vi "Cuadricula.vi"(0 "Image In":T3, 1 "ROI Descriptor (Pattern Matching 1)":T2={"Global Rectangle"=[20, 20, 1260, 700], "Contours"=[{"ID"=enum."External", "Type"=3, "Coordinates"=[20, 20, 1260, 700]}]} {"Contours"."Type" items=["No Selection", "Point", "Line", "Rectangle", "Oval", "Polygon", "Freehand Region", "Annulus", "Unused2", "Unused3", "Broken Line", "Freehand Line", "Rotated Rectangle"]}, 2 "Advanced Options (Pattern Matching 1)":cluster{"Item":T1, "Value":dbl}[](array[cluster]) {"Item" items=["LD Sampling - Minimum Constrast"=0, "LD Sampling - Enable Subpixel Accuracy"=1, "LD Sampling - Search Strategy"=2, "LD Sampling - Subpixel Iterations"=3, "LD Sampling - Subpixel Tolerance"=4, "LD Sampling - Initial Match List Length"=5, "LD Sampling - Match List Reduction Factor"=6, "LD Sampling - Initial Step Size"=7, "LD Sampling - Intermediate Angular Accuracy"=8, "-"=9, "Pyramid - Max Pyramid Level"=100, "Pyramid - Minimum Contrast"=102, "Pyramid - Enable Subpixel Accuracy"=103, "Pyramid - Subpixel Iterations"=104, "Pyramid - Subpixel Tolerance"=105, "Pyramid - Initial Match List Length"=106, "Pyramid - Match List Reduction Factor"=107, "Pyramid - Intermediate Angular Accuracy"=108, "Pyramid - Process Border Matches"=109, "Pyramid - Min Match Separation Distance"=111, "Pyramid - Min Match Separation Angle"=112, "Pyramid - Max Match Overlap"=113, "Pyramid - Max Cache in MB"=114, "Pyramid - Clear Cache"=115, "Pyramid - Enable Accurate Score Computation"=116, "Pyramid - Interpolation Method For Score Computation"=117, "Pyramid - Enable Target To Template Score"=118, "-"=119, "Enable Defect Map"=200]}, 3 "Template File Path (Pattern Matching 1)":path=path "C:/Users/cseba/OneDrive/Escritorio/Proyecto Final LabView/Cuadricula.png", 7 "error in":errorcluster) -> (20 "Image Out":T3, 21 "Matches (Pattern Matching 1)":T4(array[cluster]) {"Bounding Box"."y" format="%.2f"; "Bounding Box"."x" format="%.2f"; "Position"."y" format="%.2f"; "Position"."x" format="%.2f"; "Score" format="%.2f"; "Scale" format="%.2f"; "Angle" format="%.2f"}, 22 "Number of Matches (Pattern Matching 1)":i32, 27 "error out":errorcluster)   [LabVIEW 2024]
uses:
  <vilib>/vision/Image Controls.llb/IMAQ Image.ctl
  <vilib>/vision/Pattern Matching.llb/IMAQ Pattern Match Advanced Options.ctl
  <vilib>/vision/NI_Vision_Development_Module.lvlib
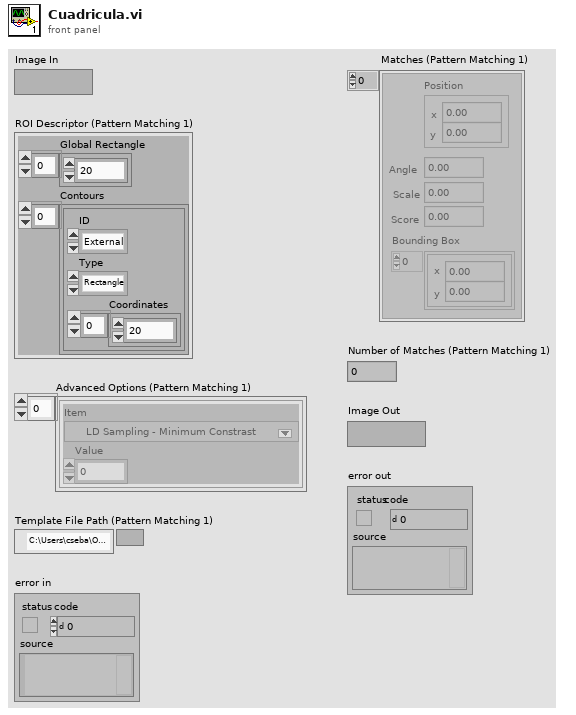
[diagram p1: front panel]
types:
  T1 = typedef "IMAQ Pattern Match Advanced Options.ctl" = u16
  T2 = cluster{"Global Rectangle":i32[], "Contours":cluster{"ID":enum32{"External", "Internal"}, "Type":u32, "Coordinates":i32[]}[]}
  T3 = typedef "IMAQ Image.ctl" = refnum<image>
  T4 = cluster{"Position":cluster{"x":sgl, "y":sgl}, "Angle":sgl, "Scale":sgl, "Score":sgl, "Bounding Box":cluster{"x":sgl, "y":sgl}[]}[]
  T5 = cluster{"Number of Matches Requested":i32, "Minimum Match Score":sgl, "Angle Ranges":cluster{"Start Angle":sgl, "End Angle":sgl}[]}
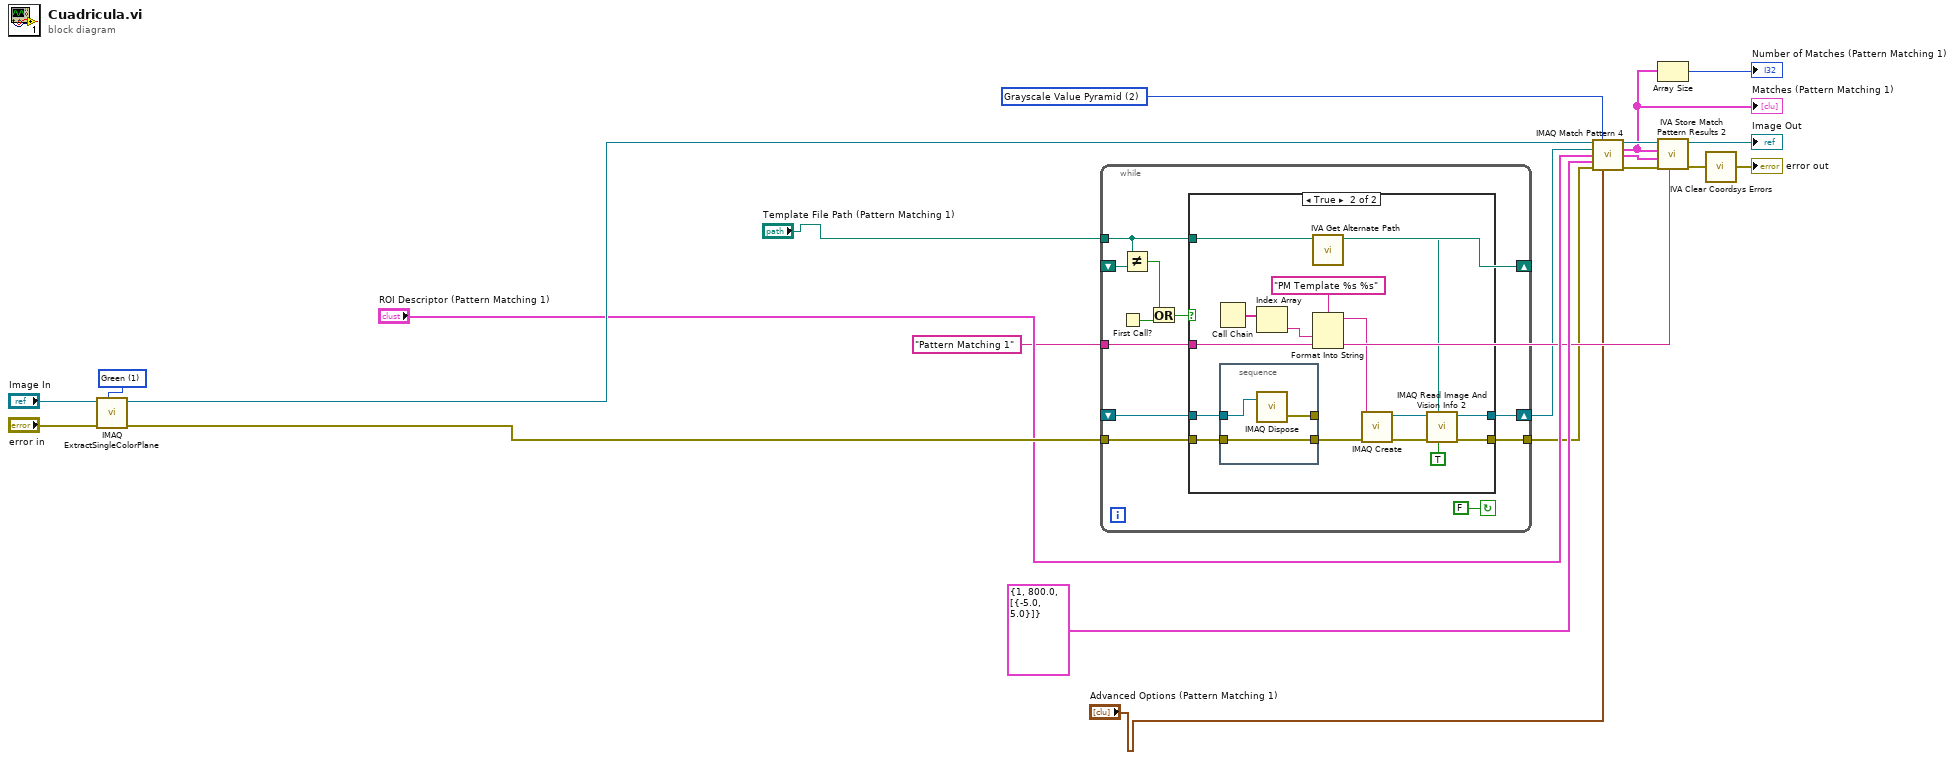
[diagram p0: block diagram]
diagram:
  w12 = 2 items=["All", "Low Discrepancy Sampling", "Grayscale Value Pyramid", "Gradients Pyramid"] ("Algorithm")
  w8 = "Pattern Matching 1" ("Step Name")
  w21 = 1 items=["Red", "Green", "Blue", "Hue", "Saturation", "Luminance", "Value", "Intensity"] ("Color Plane")
  n1 = call "IMAQ ExtractSingleColorPlane"("Color Plane"=w21, "error in (no error)"="error in", "Image Src"="Image In") -> ("error out"=w18:errorcluster, "Image Dst Out"=w16:T3)  [unwired: 1 in, 6 out]
  n2 = while {
    shift-right: [w32] -> w5
    shift-left: _ -> [w31]
    tunnel: [w29] -> w4
    tunnel: w18 -> [w28]
    tunnel: "Template File Path (Pattern Matching 1)" -> [w25]
    tunnel: w8 -> [w27]
    shift-right: [w25] -> _
    shift-left: _ -> [w26]
    stop <- FALSE continue-if-true
    n3 = First Call?() -> (First Call?: T/F=w24:bool)
    n4 = Not Equal?(x=w25, y=w26) -> (x != y?=w23:bool)
    n5 = Or(x=w23, y=w24) -> (x .or. y?=w22:bool)
    n6 = case shown="True" w22 {
      tunnel: [w34 w39] -> w32
      tunnel: w31 -> [w34 w43]
      tunnel: [w33 w40] -> w29
      tunnel: w28 -> [w33 w42]
      tunnel: w25 -> [_ w44]
      tunnel: w27 -> [_ w45]
      frame False {
      }
      frame True {
        n7 = Call Chain() -> (call chain=w47:string[])
        n8 = stacked-sequence {
          tunnel: w43 -> [w52]
          tunnel: w42 -> [w51]
          tunnel: [w51] -> w36
          tunnel: [w50] -> _
          frame #0 {
            n9 = call "IMAQ Dispose"("Image"=w52) -> ("error out"=w50:errorcluster)  [unwired: 2 in, 3 out]
          }
        }
        n10 = Index Array(array=w47) -> (element=w46:string)  [unwired: 1 in]
        n11 = call <vilib>:"IVA Get Alternate Path.vi"("Path In"=w44) -> ("Path Out"=w41:path)  [unwired: 10 out]
        n12 = Format Into String(format string="PM Template %s %s" ("Image Name"), w46, w45) -> (resulting string=w49:string)  [unwired: 2 in, 1 out]
        n13 = call "IMAQ Create"("Image Name"=w49, "error in (no error)"=w36) -> ("New Image"=w38:T3, "error out"=w37:errorcluster)  [unwired: 2 in, 1 out]
        n14 = call "IMAQ Read Image And Vision Info 2"("Use File Path Image Type"=TRUE, "File Path"=w41, "error in (no error)"=w37, "Image"=w38) -> ("error out"=w40:errorcluster, "Image Out"=w39:T3)  [unwired: 5 in, 1 out]
      }
    }
  }
  n15 = call "IMAQ Match Pattern 4"("Image"=w16, "Algorithm"=w12, "Template Image"=w5, "ROI Descriptor"="ROI Descriptor (Pattern Matching 1)", "Parameters"=T5 {"Number of Matches Requested"=1, "Minimum Match Score"=800.0, "Angle Ranges"=[{"Start Angle"=-5.0, "End Angle"=5.0}]}, "error in (no error)"=w4, "Advanced Options"="Advanced Options (Pattern Matching 1)") -> ("Image (duplicate)"=w13:T3, "Matches (pixel)"=w7:T4, "Matches (real-world)"=w6:T4, "error out"=w14:errorcluster)  [unwired: 4 in, 1 out]
  "Matches (Pattern Matching 1)" <- w7
  n16 = Array Size(array=w7) -> (size(s)=→"Number of Matches (Pattern Matching 1)":i32)
  n17 = call <vilib>:"IVA Store Match Pattern Results 2.vi"("Step Name"=w8, "error in (no error)"=w14, "Matches (real-world)"=w6, "Matches (pixel)"=w7, "Image in"=w13) -> ("error out"=w3:errorcluster, "Image dup"=→"Image Out":T3)  [unwired: 1 in, 4 out]
  n18 = call <vilib>:"IVA Clear Coordsys Errors.vi"("error in (no error)"=w3) -> ("error out"=→"error out":errorcluster)  [unwired: 10 in]
